vi "UserID.Handle.Special.Requriement.vi"(4 "error in":errorcluster, 5 "User.ID(write)":string, 6 "User.ID(original)":string, 7 "Mode":enum16{"Write", "Read"}(ring)=enum."Read") -> (0 "error out":errorcluster, 3 "User.ID(read)":string)   [LabVIEW 2020]
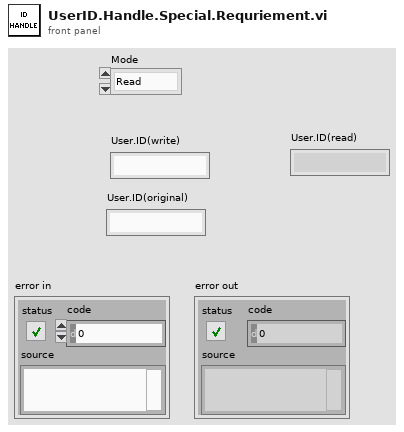
[diagram p1: front panel]
types:
  T1 = enum16{"open", "replace", "create", "open or create", "replace or create", "replace or create with confirmation"}
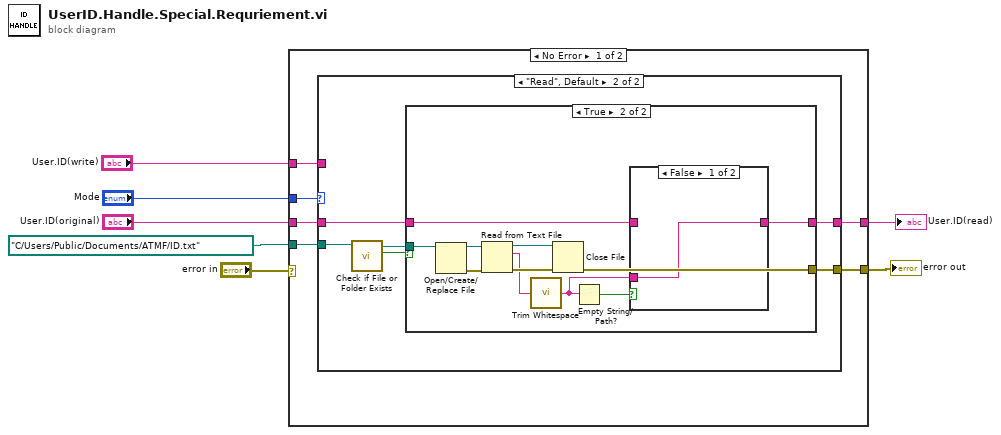
[diagram p0: block diagram]
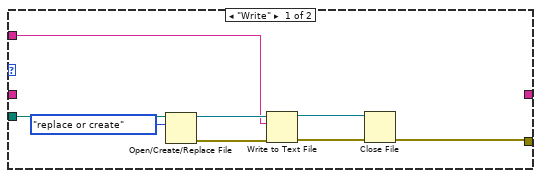
[diagram p2: hidden frame]
diagram:
  n1 = case shown="No Error" "error in" {
    selector: "error in" -> [_ w42]
    tunnel: "Mode" -> [w13 _]
    tunnel: path "C:/Users/Public/Documents/ATMF/ID.txt" -> [w12 _]
    tunnel: [w11 w42] -> w4
    tunnel: "User.ID(write)" -> [w10 _]
    tunnel: [w9 _] -> w2
    tunnel: "User.ID(original)" -> [w8 _]
    frame No Error {
      n2 = case shown="\"Read\", Default" w13 {
        tunnel: w12 -> [w17 w27]
        tunnel: [w15 w25] -> w11
        tunnel: w10 -> [w14 _]
        tunnel: [_ w23] -> w9
        tunnel: w8 -> [_ w22]
        frame "Write" {
          n3 = Open/Create/Replace File(file path (use dialog)=w17, operation (0:open)=T1."replace or create") -> (refnum out=w19:refnum<file>, error out=w21:errorcluster)  [unwired: 4 in, 1 out]
          n4 = Write to Text File(file (use dialog)=w19, text=w14, error in=w21) -> (refnum out=w18:refnum<file>, error out=w20:errorcluster)  [unwired: 1 in, 1 out]
          n5 = Close File(refnum=w18, error in=w20) -> (error out=w15:errorcluster)  [unwired: 1 out]
        }
        frame "Read", Default {
          n6 = call <vilib>:"Check if File or Folder Exists.vi"("path"=w27) -> ("file or folder exists?"=w26:bool, "dup path"=w24:path)  [unwired: 8 in, 1 out]
          n7 = case shown="True" w26 {
            tunnel: [_ w35] -> w25
            tunnel: w24 -> [_ w34]
            tunnel: [w28 w31] -> w23
            tunnel: w22 -> [w28 w30]
            frame False {
            }
            frame True {
              n8 = Open/Create/Replace File(file path (use dialog)=w34) -> (refnum out=w37:refnum<file>, error out=w39:errorcluster)  [unwired: 5 in, 1 out]
              n9 = Read from Text File(file (use dialog)=w37, error in=w39) -> (refnum out=w36:refnum<file>, text=w33:string, error out=w38:errorcluster)  [unwired: 2 in, 1 out]
              n10 = call <vilib>:"Trim Whitespace.vi"("string"=w33) -> ("trimmed string"=w29:string)  [unwired: 1 in]
              n11 = Close File(refnum=w36, error in=w38) -> (error out=w35:errorcluster)  [unwired: 1 out]
              n12 = Empty String/Path?(string/path=w29) -> (empty?=w32:bool)
              n13 = case shown="False" w32 {
                tunnel: [w40 w41] -> w31
                tunnel: w30 -> [_ w41]
                tunnel: w29 -> [w40 _]
                frame False {
                }
                frame True {
                }
              }
            }
          }
        }
      }
    }
    frame Error {
    }
  }
  "error out" <- w4
  "User.ID(read)" <- w2
